vi "Joystick_Var.vi"() -> (0 "JoyStick":T3)   [LabVIEW 2015]
uses:
  <vilib>/Rock Robotics/WPI/DriverStation/WPI_DriverStationRobotMode2.ctl
  <vilib>/Rock Robotics/WPI/Camera/WPI_CameraImageSize.ctl
  Global_Var/JoyStick_Global.vi
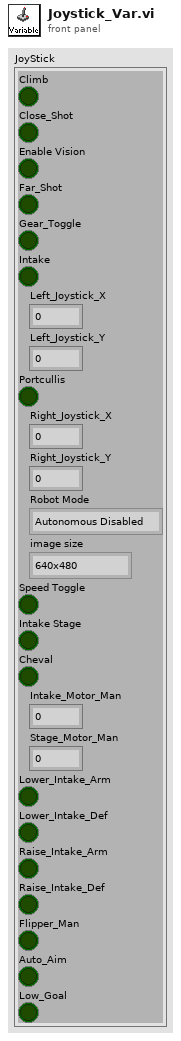
[diagram p1: front panel]
types:
  T1 = typedef "WPI_DriverStationRobotMode2.ctl" = enum16{"Autonomous Disabled", "Autonomous Enabled", "Teleop Disabled", "Teleop Enabled", "Disconnected", "Finish", "Test Disabled", "Test Enabled", "Emergency Stopped"}
  T2 = typedef "WPI_CameraImageSize.ctl" = enum16{"640x480", "320x240", "160x120", "Custom"}
  T3 = cluster{"Climb":bool, "Close_Shot":bool, "Enable Vision":bool, "Far_Shot":bool, "Gear_Toggle":bool, "Intake":bool, "Left_Joystick_X":dbl, "Left_Joystick_Y":dbl, "Portcullis":bool, "Right_Joystick_X":dbl, "Right_Joystick_Y":dbl, "Robot Mode":T1, "image size":T2, "Speed Toggle":bool, "Intake Stage":bool, "Cheval":bool, "Intake_Motor_Man":dbl, "Stage_Motor_Man":dbl, "Lower_Intake_Arm":bool, "Lower_Intake_Def":bool, "Raise_Intake_Arm":bool, "Raise_Intake_Def":bool, "Flipper_Man":bool, "Auto_Aim":bool, "Low_Goal":bool}
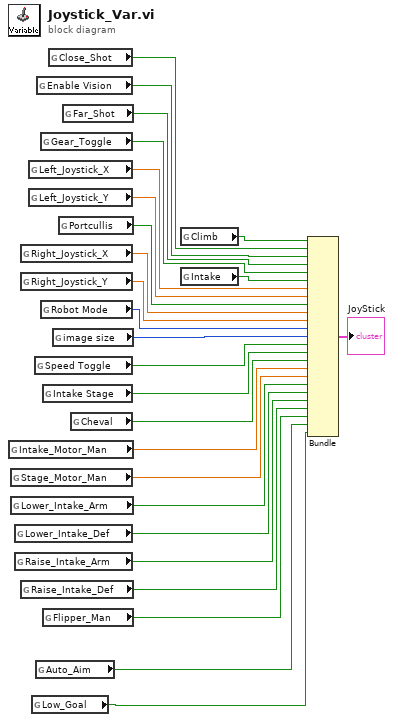
[diagram p0: block diagram]
diagram:
  n1 = global read "JoyStick_Global.vi" "Intake_Motor_Man"() -> (w10:dbl)
  n2 = global read "JoyStick_Global.vi" "Stage_Motor_Man"() -> (w9:dbl)
  n3 = global read "JoyStick_Global.vi" "Lower_Intake_Arm"() -> (w8:bool)
  n4 = global read "JoyStick_Global.vi" "Lower_Intake_Def"() -> (w7:bool)
  n5 = global read "JoyStick_Global.vi" "Raise_Intake_Arm"() -> (w6:bool)
  n6 = global read "JoyStick_Global.vi" "Right_Joystick_X"() -> (w17:dbl)
  n7 = global read "JoyStick_Global.vi" "Right_Joystick_Y"() -> (w16:dbl)
  n8 = global read "JoyStick_Global.vi" "Raise_Intake_Def"() -> (w5:bool)
  n9 = global read "JoyStick_Global.vi" "Left_Joystick_X"() -> (w20:dbl)
  n10 = global read "JoyStick_Global.vi" "Left_Joystick_Y"() -> (w19:dbl)
  n11 = global read "JoyStick_Global.vi" "Low_Goal"() -> (w2:bool)
  n12 = global read "JoyStick_Global.vi" "Speed Toggle"() -> (w13:bool)
  n13 = global read "JoyStick_Global.vi" "Auto_Aim"() -> (w3:bool)
  n14 = global read "JoyStick_Global.vi" "Enable Vision"() -> (w24:bool)
  n15 = global read "JoyStick_Global.vi" "Gear_Toggle"() -> (w22:bool)
  n16 = global read "JoyStick_Global.vi" "Robot Mode"() -> (w15:T1)
  n17 = global read "JoyStick_Global.vi" "Intake Stage"() -> (w12:bool)
  n18 = global read "JoyStick_Global.vi" "Flipper_Man"() -> (w4:bool)
  n19 = global read "JoyStick_Global.vi" "Close_Shot"() -> (w25:bool)
  n20 = global read "JoyStick_Global.vi" "image size"() -> (w14:T2)
  n21 = global read "JoyStick_Global.vi" "Portcullis"() -> (w18:bool)
  n22 = global read "JoyStick_Global.vi" "Far_Shot"() -> (w23:bool)
  n23 = global read "JoyStick_Global.vi" "Cheval"() -> (w11:bool)
  n24 = global read "JoyStick_Global.vi" "Climb"() -> (w26:bool)
  n25 = global read "JoyStick_Global.vi" "Intake"() -> (w21:bool)
  n26 = Bundle("Climb"=w26, "Close_Shot"=w25, "Enable Vision"=w24, "Far_Shot"=w23, "Gear_Toggle"=w22, "Intake"=w21, "Left_Joystick_X"=w20, "Left_Joystick_Y"=w19, "Portcullis"=w18, "Right_Joystick_X"=w17, "Right_Joystick_Y"=w16, "Robot Mode"=w15, "image size"=w14, "Speed Toggle"=w13, "Intake Stage"=w12, "Cheval"=w11, "Intake_Motor_Man"=w10, "Stage_Motor_Man"=w9, "Lower_Intake_Arm"=w8, "Lower_Intake_Def"=w7, "Raise_Intake_Arm"=w6, "Raise_Intake_Def"=w5, "Flipper_Man"=w4, "Auto_Aim"=w3, "Low_Goal"=w2) -> (→"JoyStick":T3)  [unwired: 1 in]
